vi "纳清蓝绿藻_所有参数读取.vi"(8 "error in (no error)":errorcluster caption="错误输入（无错误）", 11 "MB session in":refnum<class "MB_Master.lvclass">) -> (0 "error out":errorcluster caption="错误输出", 2 "输出值":T1 {"波特率" items=["4800", "9600", "19200", "38400", "57600", "115200"]}, 3 "MB session out":refnum<class "MB_Master.lvclass">)   [LabVIEW 2016, in "斯坦道多参数.lvlib"]
uses:
  <vilib>/Plasmionique/MB Master/MB_Master/MB_Master.lvclass
  <vilib>/Plasmionique/MB Master/MB Master.lvlib
  <vilib>/ptbypt/NI_PtbyPt.lvlib
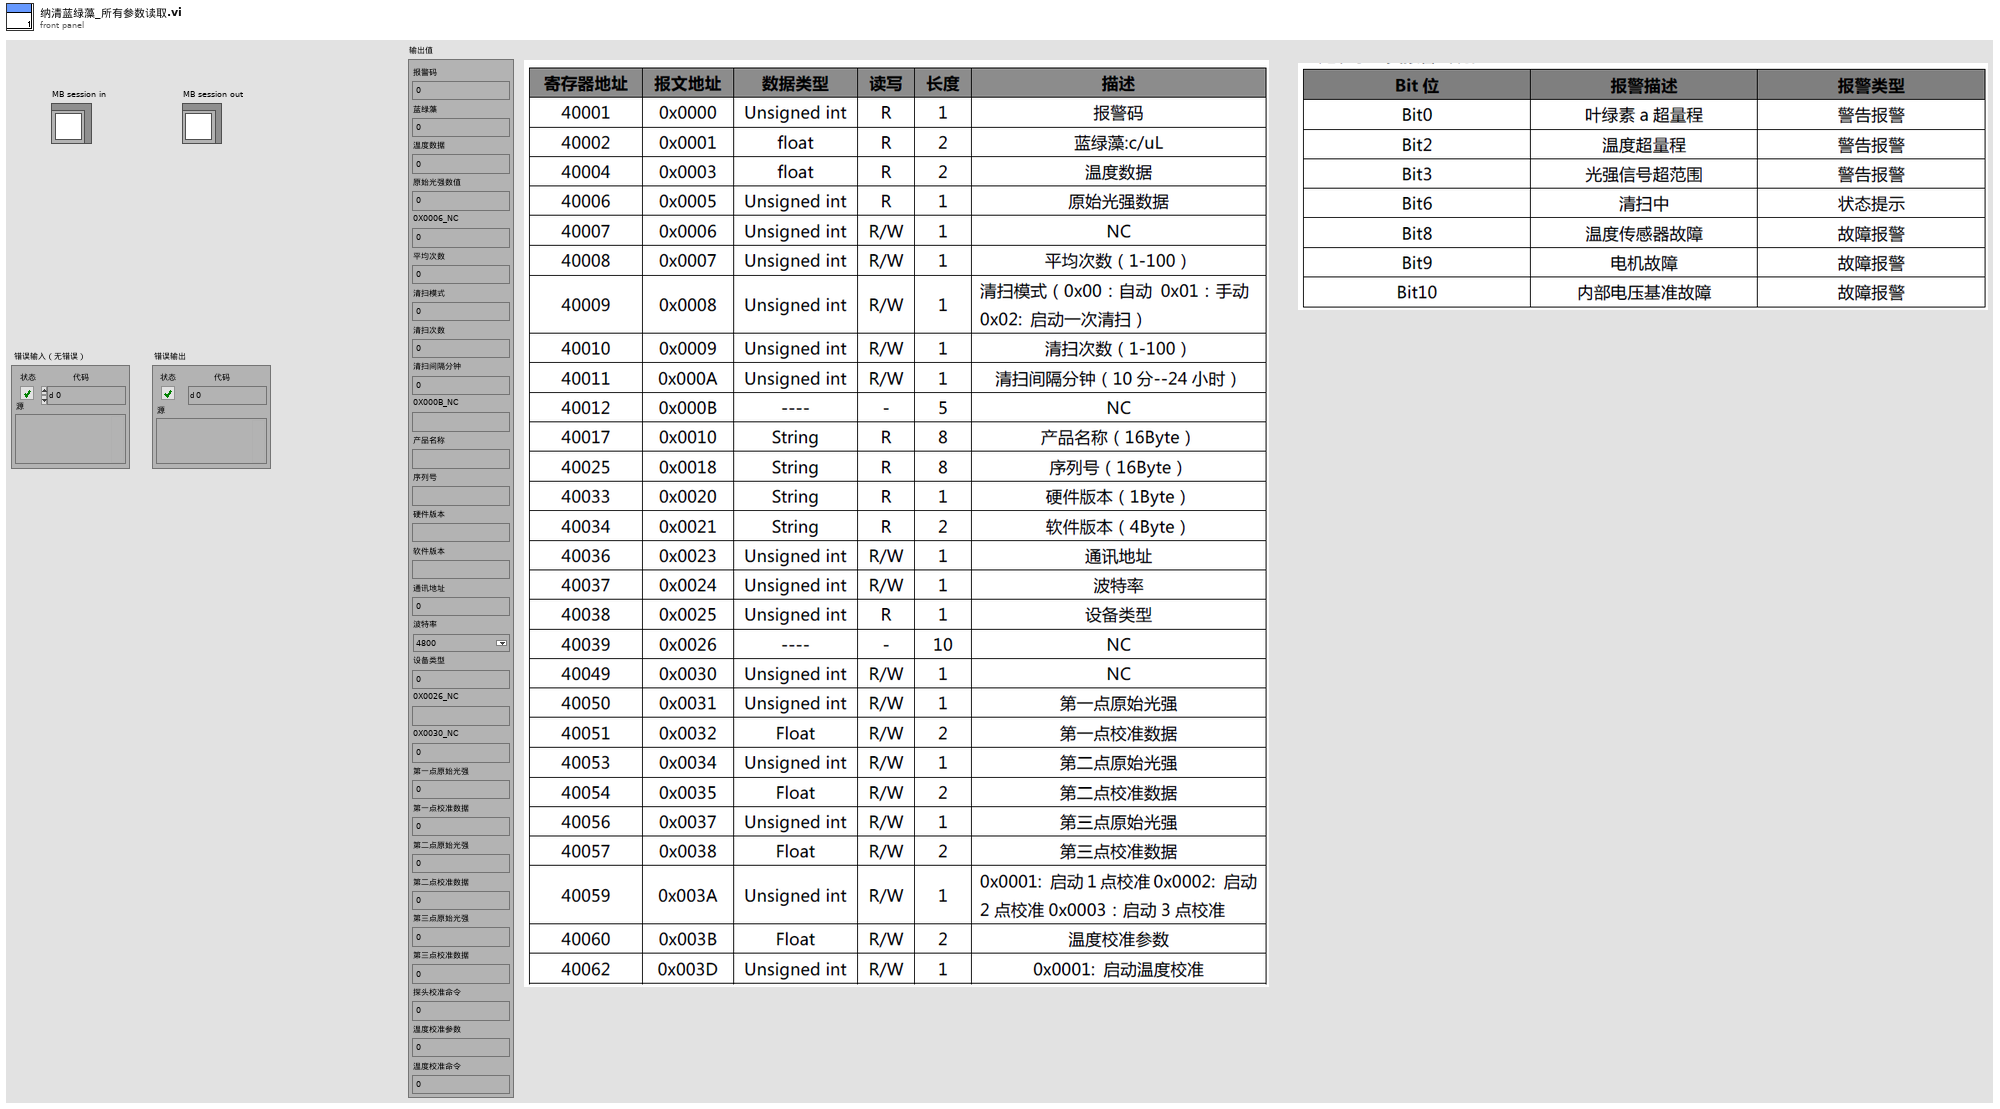
[diagram p1: front panel]
types:
  T1 = cluster{"报警码":u16, "蓝绿藻":sgl, "温度数据":sgl, "原始光强数值":u16, "0X0006_NC":u16, "平均次数":u16, "清扫模式":u16, "清扫次数":u16, "清扫间隔分钟":u16, "0X000B_NC":string, "产品名称":string, "序列号":string, "硬件版本":string, "软件版本":string, "通讯地址":u16, "波特率":u16, "设备类型":u16, "0X0026_NC":string, "0X0030_NC":u16, "第一点原始光强":u16, "第一点校准数据":sgl, "第二点原始光强":u16, "第二点校准数据":sgl, "第三点原始光强":u16, "第三点校准数据":sgl, "探头校准命令":u16, "温度校准参数":sgl, "温度校准命令":u16}
  T2 = cluster{u16, "Filtered x":dbl, "数值":sgl, u16, u16, u16, u16, u16, u16, "类型":string, "类型":string, "类型":string, "类型":string, "类型":string, u16, u16, u16, "类型":string, u16, u16, "数值":sgl, u16, "数值":sgl, u16, "数值":sgl, u16, "数值":sgl, u16}
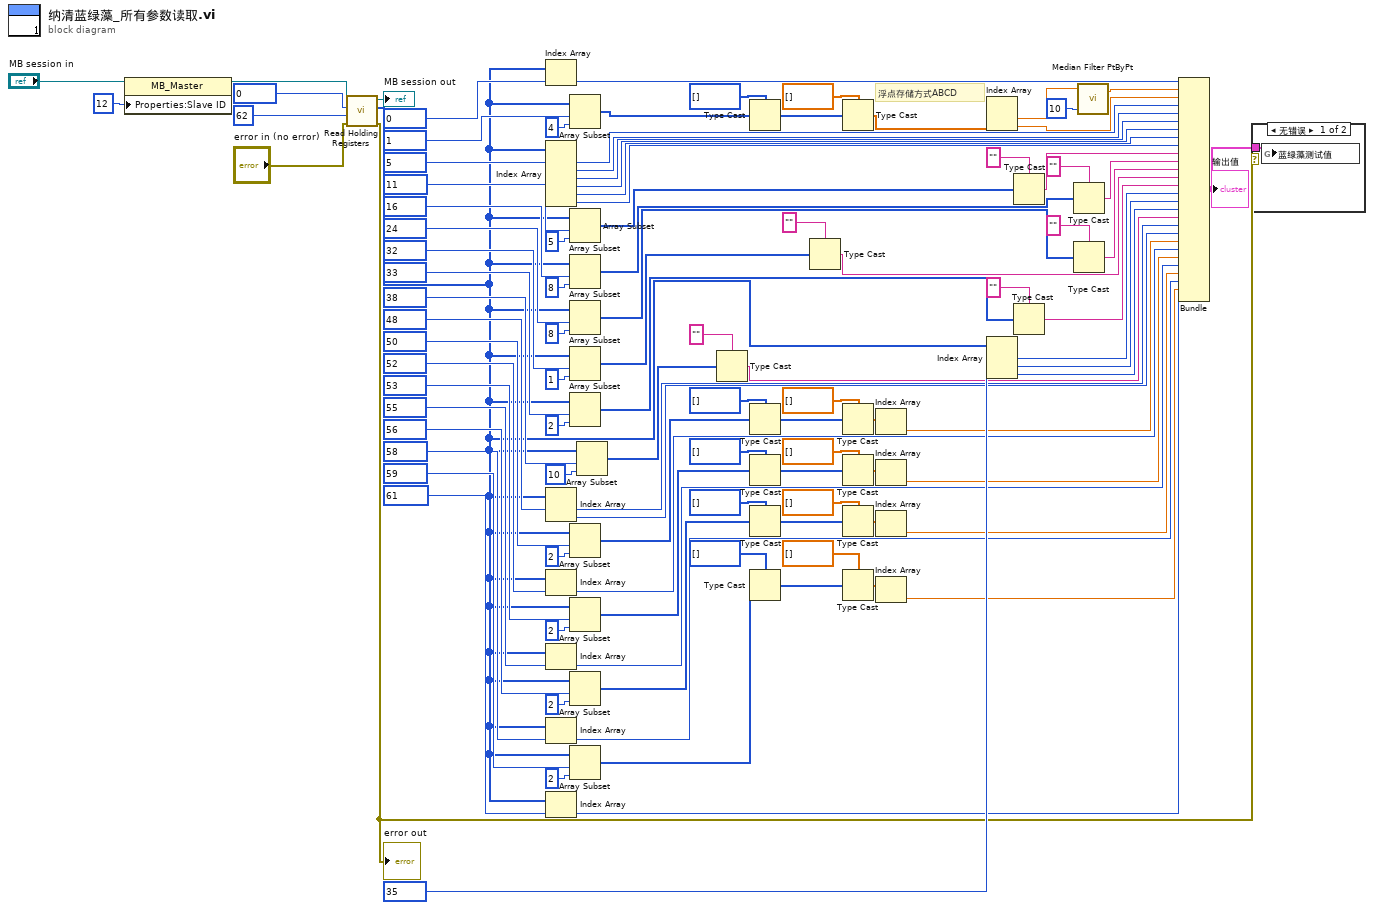
[diagram p0: block diagram]
diagram:
  # "浮点存储方式ABCD"
  n1 = property class="MB_Master"(reference="MB session in", "Properties:Slave ID"=u8 12 ("Slave ID")) -> (reference out=w97:refnum<class "MB_Master.lvclass">)  [unwired: 1 in, 1 out]
  n2 = call <vilib>:"Read Holding Registers.vi"("error in (no error)"="error in (no error)", "quantity"=u16 62, "starting address"=u16 0, "MB session in"=w97) -> ("error out"=w8:errorcluster, "Registers"=w10:u16[], "MB session out"=→"MB session out":refnum<class "MB_Master.lvclass">)  [unwired: 5 in]
  "error out" <- w8
  n3 = Index Array(array=w10, index=u16 0 ("starting address")) -> (element=w105:u16)
  n4 = Index Array(array=w10, index #1=u16 5 ("starting address")) -> (element #1=w92:u16, element #2=w91:u16, element #3=w90:u16, element #4=w89:u16, element #5=w88:u16, element #6=w87:u16)  [unwired: 5 in]
  n5 = Index Array(array=w10, index #1=u16 48 ("starting address")) -> (element #1=w51:u16, element #2=w50:u16)  [unwired: 1 in]
  n6 = Index Array(array=w10, index=u16 52 ("starting address")) -> (element=w33:u16)
  n7 = Index Array(array=w10, index=u16 55 ("starting address")) -> (element=w23:u16)
  n8 = Index Array(array=w10, index=u16 58 ("starting address")) -> (element=w13:u16)
  n9 = Index Array(array=w10, index=u16 61 ("starting address")) -> (element=w9:u16)
  n10 = Array Subset(array=w10, index=u16 1 ("starting address"), length=4 ("长度")) -> (w101:u16[])
  n11 = Array Subset(array=w10, index=u16 11 ("starting address"), length=5 ("长度")) -> (w84:u16[])
  n12 = Array Subset(array=w10, index=u16 16 ("starting address"), length=8 ("长度")) -> (w80:u16[])
  n13 = Array Subset(array=w10, index=u16 24 ("starting address"), length=8 ("长度")) -> (w74:u16[])
  n14 = Array Subset(array=w10, index=u16 32 ("starting address"), length=1 ("长度")) -> (w70:u16[])
  n15 = Array Subset(array=w10, index=u16 33 ("starting address"), length=2 ("长度")) -> (w64:u16[])
  n16 = Array Subset(array=w10, index=u16 50 ("starting address"), length=2 ("长度")) -> (w48:u16[])
  n17 = Array Subset(array=w10, index=u16 53 ("starting address"), length=2 ("长度")) -> (w36:u16[])
  n18 = Array Subset(array=w10, index=u16 56 ("starting address"), length=2 ("长度")) -> (w29:u16[])
  n19 = Array Subset(array=w10, index=u16 59 ("starting address"), length=2 ("长度")) -> (w16:u16[])
  n20 = Array Subset(array=w10, index=u16 38 ("starting address"), length=10 ("长度")) -> (w54:u16[])
  n21 = Type Cast(type="" ("类型"), x=w54) -> (*(type *) &x=w53:string)
  n22 = Type Cast(type=u32[] [] ("数组 2"), x=w101) -> (*(type *) &x=w7:u32[])
  n23 = Type Cast(type=u32[] [] ("数组 2"), x=w48) -> (*(type *) &x=w46:u32[])
  n24 = Type Cast(type=u32[] [] ("数组 2"), x=w36) -> (*(type *) &x=w38:u32[])
  n25 = Type Cast(type=u32[] [] ("数组 2"), x=w29) -> (*(type *) &x=w27:u32[])
  n26 = Type Cast(type=u32[] [] ("数组 2"), x=w16) -> (*(type *) &x=w18:u32[])
  n27 = Type Cast(type="" ("类型"), x=w70) -> (*(type *) &x=w67:string)
  n28 = Type Cast(type=sgl[] [] ("数组 2"), x=w7) -> (*(type *) &x=w100:sgl[])
  n29 = Type Cast(type=sgl[] [] ("数组 2"), x=w46) -> (*(type *) &x=w43:sgl[])
  n30 = Type Cast(type=sgl[] [] ("数组 2"), x=w38) -> (*(type *) &x=w41:sgl[])
  n31 = Type Cast(type=sgl[] [] ("数组 2"), x=w27) -> (*(type *) &x=w24:sgl[])
  n32 = Type Cast(type=sgl[] [] ("数组 2"), x=w18) -> (*(type *) &x=w21:sgl[])
  n33 = Index Array(array=w43) -> (element=w42:sgl)  [unwired: 1 in]
  n34 = Index Array(array=w41) -> (element=w32:sgl)  [unwired: 1 in]
  n35 = Index Array(array=w24) -> (element=w22:sgl)  [unwired: 1 in]
  n36 = Index Array(array=w21) -> (element=w12:sgl)  [unwired: 1 in]
  n37 = Index Array(array=w100) -> (element #1=w2:sgl, element #2=w95:sgl)  [unwired: 2 in]
  n38 = Index Array(array=w10, index #1=u16 35 ("starting address")) -> (element #1=w60:u16, element #2=w59:u16, element #3=w58:u16)  [unwired: 2 in]
  n39 = Type Cast(type="" ("类型"), x=w84) -> (*(type *) &x=w82:string)
  n40 = Type Cast(type="" ("类型"), x=w64) -> (*(type *) &x=w62:string)
  n41 = Type Cast(type="" ("类型"), x=w80) -> (*(type *) &x=w77:string)
  n42 = Type Cast(type="" ("类型"), x=w74) -> (*(type *) &x=w72:string)
  n43 = call <vilib>:"Median Filter PtByPt.vi"("rank"=10, "x"=w2) -> ("Filtered x"=w1:dbl)  [unwired: 2 in, 1 out]
  n44 = Bundle(w105, "Filtered x"=w1, "数值"=w95, w92, w91, w90, w89, w88, w87, "类型"=w82, "类型"=w77, "类型"=w72, "类型"=w67, "类型"=w62, w60, w59, w58, "类型"=w53, w51, w50, "数值"=w42, w33, "数值"=w32, w23, "数值"=w22, w13, "数值"=w12, w9) -> (w4:T2)  [unwired: 1 in]
  "输出值" <- w4
  n45 = case shown="无错误" w8 {
    tunnel: w4 -> [w108 _]
    frame No Error {
      n46 = global write "纳清过程全局变量.vi" "蓝绿藻测试值"(w108) -> ()
    }
    frame Error {
    }
  }
